vi "Build DashBoard Data.vi"(9 "All_Outputs":T7, 10 "All_Sensor_Readings":T10, 11 "All Driver Commands":T4) -> ()   [LabVIEW 2012]
doc: "This VI builds data and sends it back to the dashboard PC program. By default it sends back the raw values for the first analog, digital, and solenoid module. Modify it to send back the data you want to view. Consider adding higher level data to the Dashboard Datatype.ctl and to this VI. Then update the Dashboard to display the data however you like.\n\nThis software is licensed. Open the labview\\readme\\WPI Robotics Library Open Source License.txt file for more information."
uses:
  All_Commands.ctl
  Cirular Shooter/circular_shooter_commands.ctl
  Climber/Climber_Commands.ctl
  All_Outputs.ctl
  Cirular Shooter/Shooter_Outputs.ctl
  Climber/Climber_Outputs.ctl
  All_Sensor_Readings.ctl
  Climber/climber_sensor_readings.ctl
  Cirular Shooter/Shooter_inputs.ctl
  Field Drive/Field_Drive_out.ctl
  Dashboard Datatype.ctl
  Joystick_Inputs.ctl
  <vilib>/Rock Robotics/WPI/Joystick/WPI_JoystickButtonState.ctl
panel:
  in  "Joystick_Inputs":T1
  out "Dashboard Data":T3
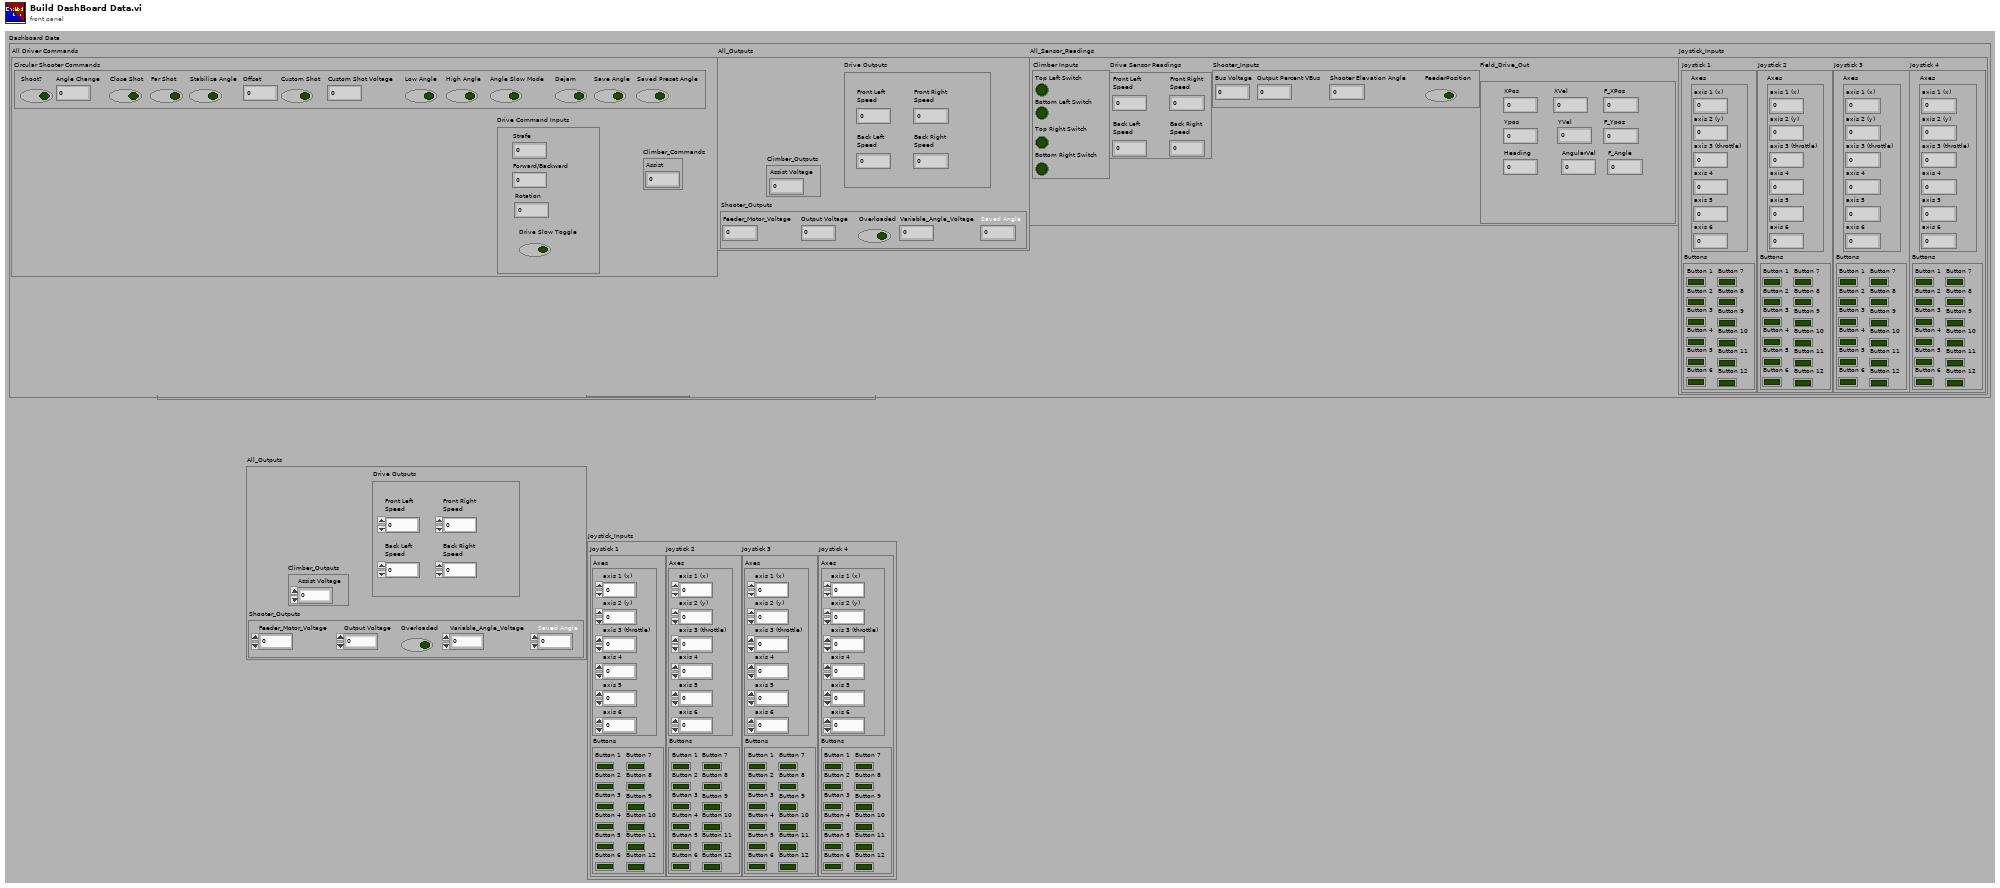
[diagram p1: front panel]
types:
  T1 = typedef "Joystick_Inputs.ctl" = cluster{"Joystick 1":cluster{"Axes":cluster{"axis 1 (x)":dbl, "axis 2 (y)":dbl, "axis 3 (throttle)":dbl, "axis 4":dbl, "axis 5":dbl, "axis 6":dbl}, "Buttons":T2}, "Joystick 2":cluster{"Axes":cluster{"axis 1 (x)":dbl, "axis 2 (y)":dbl, "axis 3 (throttle)":dbl, "axis 4":dbl, "axis 5":dbl, "axis 6":dbl}, "Buttons":T2}, "Joystick 3":cluster{"Axes":cluster{"axis 1 (x)":dbl, "axis 2 (y)":dbl, "axis 3 (throttle)":dbl, "axis 4":dbl, "axis 5":dbl, "axis 6":dbl}, "Buttons":T2}, "Joystick 4":cluster{"Axes":cluster{"axis 1 (x)":dbl, "axis 2 (y)":dbl, "axis 3 (throttle)":dbl, "axis 4":dbl, "axis 5":dbl, "axis 6":dbl}, "Buttons":T2}}
  T2 = typedef "WPI_JoystickButtonState.ctl" = cluster{"Button 1":bool, "Button 2":bool, "Button 3":bool, "Button 4":bool, "Button 5":bool, "Button 6":bool, "Button 7":bool, "Button 8":bool, "Button 9":bool, "Button 10":bool, "Button 11":bool, "Button 12":bool}
  T3 = typedef "Dashboard Datatype.ctl" = cluster{"All Driver Commands":T4, "All_Outputs":T7, "All_Sensor_Readings":T10, "Joystick_Inputs ":T1}
  T4 = typedef "All_Commands.ctl" = cluster{"Circular Shooter Commands":T5, "Drive Command Inputs":cluster{"Strafe":dbl, "Forward/Backward":dbl, "Rotation":dbl, "Drive Slow Toggle":bool}, "Climber_Commands":T6}
  T5 = typedef "circular_shooter_commands.ctl" = cluster{"Shoot?":bool, "Angle Change":dbl, "Close Shot":bool, "Far Shot":bool, "Stabilize Angle ":bool, "Offset":dbl, "Custom Shot":bool, "Custom Shot Voltage":dbl, "Low Angle":bool, "High Angle":bool, "Angle Slow Mode":bool, "Dejam":bool, "Save Angle":bool, "Saved Preset Angle":bool}
  T6 = typedef "Climber_Commands.ctl" = cluster{"Assist":dbl}
  T7 = typedef "All_Outputs.ctl" = cluster{"Drive Outputs":cluster{"Front Left\nSpeed":dbl, "Back Left\nSpeed":dbl, "Front Right\nSpeed":dbl, "Back Right\nSpeed":dbl}, "Shooter_Outputs":T8, "Climber_Outputs":T9}
  T8 = typedef "Shooter_Outputs.ctl" = cluster{"Feeder_Motor_Voltage":dbl, "Output Voltage":dbl, "Overloaded":bool, "Variable_Angle_Voltage":dbl, "Saved Angle":dbl}
  T9 = typedef "Climber_Outputs.ctl" = cluster{"Assist Voltage":dbl}
  T10 = typedef "All_Sensor_Readings.ctl" = cluster{"Climber Inputs":T11, "Drive Sensor Readings":cluster{"Front Left\nSpeed":dbl, "Back Left\nSpeed":dbl, "Front Right\nSpeed":dbl, "Back Right\nSpeed":dbl}, "Shooter_Inputs":T12, "Field_Drive_Out\n":T13}
  T11 = typedef "climber_sensor_readings.ctl" = cluster{"Top Left Switch":bool, "Bottom Left Switch":bool, "Top Right Switch":bool, "Bottom Right Switch":bool}
  T12 = typedef "Shooter_inputs.ctl" = cluster{"Bus Voltage":dbl, "Output Percent VBus":dbl, "Shooter Elevation Angle":dbl, "FeederPosition":bool}
  T13 = typedef "Field_Drive_out.ctl" = cluster{"XPos":dbl, "Ypos":dbl, "XVel":dbl, "YVel":dbl, "Heading":dbl, "AngularVel":dbl, "F_XPos":dbl, "F_Ypos":dbl, "F_Angle":dbl}
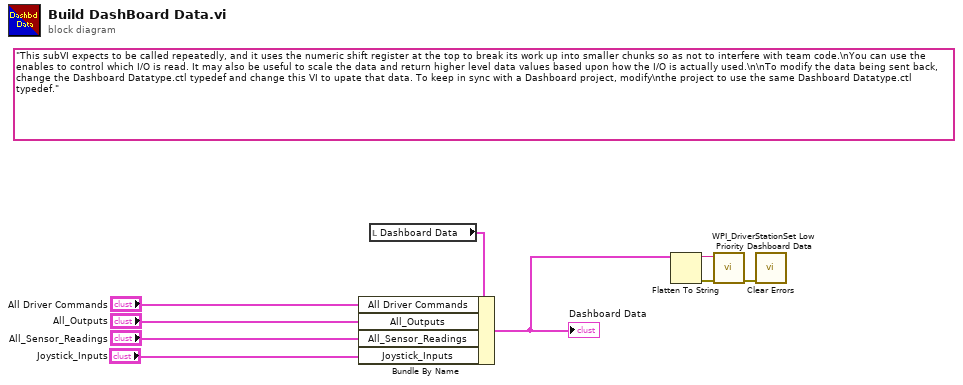
[diagram p0: block diagram]
diagram:
  (unwired) "This subVI expects to be called repeatedly, and it uses the numeric shift register at the top to break its work up into smaller chunks so as not to interfere with team code.\nYou can use the enables to control which I/O is read. It may also be useful to scale the data and return higher level data values based upon how the I/O is actually used.\n\nTo modify the data being sent back, change the Dashboard Datatype.ctl typedef and change this VI to upate that data. To keep in sync with a Dashboard project, modify\nthe project to use the same Dashboard Datatype.ctl typedef."
  n1 = local read "Dashboard Data"() -> (w9:T3)
  n2 = Bundle By Name(cluster=w9, "All Driver Commands"="All Driver Commands", "All_Outputs"="All_Outputs", "All_Sensor_Readings"="All_Sensor_Readings", "Joystick_Inputs"="Joystick_Inputs") -> (w2:T3)
  "Dashboard Data" <- w2
  n3 = Flatten To String(anything=w2) -> (data string=w3:string, error out=w4:errorcluster)  [unwired: 3 in, 1 out]
  n4 = call <vilib>:"WPI_DriverStationSet Low Priority Dashboard Data.vi"("error in (no error)"=w4, "User Data"=w3) -> ("error out"=w1:errorcluster)  [unwired: 9 in]
  n5 = call <vilib>:"Clear Errors.vi"("error in (no error)"=w1) -> ()  [unwired: 6 in, 1 out]
